vi "TCS Command Test Program.vi"() -> ()   [LabVIEW 2022 SP3]
uses:
  typedefs/CC cluster Object.ctl
  typedefs/CC cluster sidereal rate.ctl
  typedefs/CC cluster RA and DEC.ctl
  typedefs/cc cluster muRA muDEC.ctl
  Telescope/CC cluster Telescope Offsets.ctl
  TCS/TCS_external_interfaces/TCSDataDefinitions/TCSCommand/TCSTcsCommand/TCSTcsCommand.lvclass
  TCS/TCS_external_interfaces/TCSDataDefinitions/TCSCommand/TargetConfiguration/Target/FixedTarget/RADecParameters/RADecParameters.lvclass
  TCS/TCS_external_interfaces/TCSDataDefinitions/TCSCommand/TargetConfiguration/Target/FixedTarget/Declination/Declination.lvclass
  TCS/TCS_external_interfaces/TCSDataDefinitions/TCSPublicStatus/CurrentTimes/ClockTimes/ClockTimes.lvclass
  TCS/TCS_external_interfaces/TCSDataDefinitions/TCSCommand/TargetConfiguration/ScienceTargetConfiguration/ScienceTargetConfiguration.lvclass
  C:/Development/TCS/TCS_external_interfaces/TCSDataDefinitions/TCSCommand/TargetConfiguration/TargetConfiguration/TargetConfiguration.lvclass
  TCS/TCS_external_interfaces/TCSDataDefinitions/TCSCommand/TargetConfiguration/Target/FixedTarget/RADecTarget/RADecTarget.lvclass
  C:/Development/TCS/TCS_external_interfaces/TCSDataDefinitions/TCSCommand/TargetConfiguration/Target/FixedTarget/FixedTarget/FixedTarget.lvclass
  C:/Development/TCS/TCS_external_interfaces/TCSDataDefinitions/TCSCommand/TargetConfiguration/Target/Target/Target.lvclass
  TCS/TCS_external_interfaces/TCSDataDefinitions/TCSCommand/TargetConfiguration/Target/FixedTarget/Declination/Declination.lvclass/Declination.ctl
  TCS/TCS_external_interfaces/TCSDataDefinitions/TCSPublicStatus/CurrentTimes/ClockTimes/ClockTimes.lvclass/ClockTimes.ctl
  TCS/TCS_external_interfaces/TCSDataDefinitions/TCSCommand/TargetConfiguration/Target/FixedTarget/RADecParameters/RADecParameters.lvclass/RADecParameters.ctl
  TCS/TCS_external_interfaces/TCSDataDefinitions/TCSCommand/TargetConfiguration/Target/FixedTarget/RADecTarget/RADecTarget.lvclass/RADecTarget.ctl
  TCS/TCS_external_interfaces/TCSDataDefinitions/TCSCommand/TargetConfiguration/Target/FixedTarget/FixedTarget/FixedTarget.lvclass/FixedTarget.ctl
  TCS/TCS_external_interfaces/TCSDataDefinitions/TCSCommand/TargetConfiguration/TargetConfiguration/TargetConfiguration.lvclass/TargetConfiguration.ctl
  TCS/TCS_external_interfaces/TCSDataDefinitions/TCSCommand/TargetConfiguration/TargetConfiguration/TargetConfiguration.lvclass
  TCS/TCS_external_interfaces/TCSDataDefinitions/TCSCommand/TargetConfiguration/Target/FixedTarget/FixedTarget/FixedTarget.lvclass
panel:
  out "XMLout":string
  out "XML out 2":string
  in  "Object out":T1
  in  "ClassLabel":string="TCSTcsCommand"
  out "XML out":string=" <target class=\"TCSDataDefinitions.TCSCommand.TargetConfiguration.Target.FixedTarget.RADecTarget\">\n  <commandID>100</commandID>\n  <tcsErrorResponse>\r\n    <status>false</status>\r\n    <code>0</code>\r\n    <source/>\r\n  </tcsErrorResponse>\n    <raDecParameters>\n      <declination>\n        <degreesDec>0</degreesDec>\n        <minutesArc>0</minutesArc>\n        <secondsArc>0</secondsArc>\n      </declination>\n      <equinoxPrefix>B</equinoxPrefix>\n      <equinoxYear>2000</equinoxYear>\n      <frame>FK4</frame>\n      <ra>\n        <hours>0</hours>\n        <minutesTime>0</minutesTime>\n        <secondsTime>0</secondsTime>\n      </ra>\n    </raDecParameters>\n    <parallax_Arcsec>0</parallax_Arcsec>\n    <properMotion>\n      <epochPM_Yr>2009</epochPM_Yr>\n      <pmdec_ArcsPYr>0</pmdec_ArcsPYr>\n      <pmra_SPYr>0</pmra_SPYr>\n    </properMotion>\n    <rv_kps>0</rv_kps>\n    <targetName>TargetName</targetName>\n    \n</target>\n"
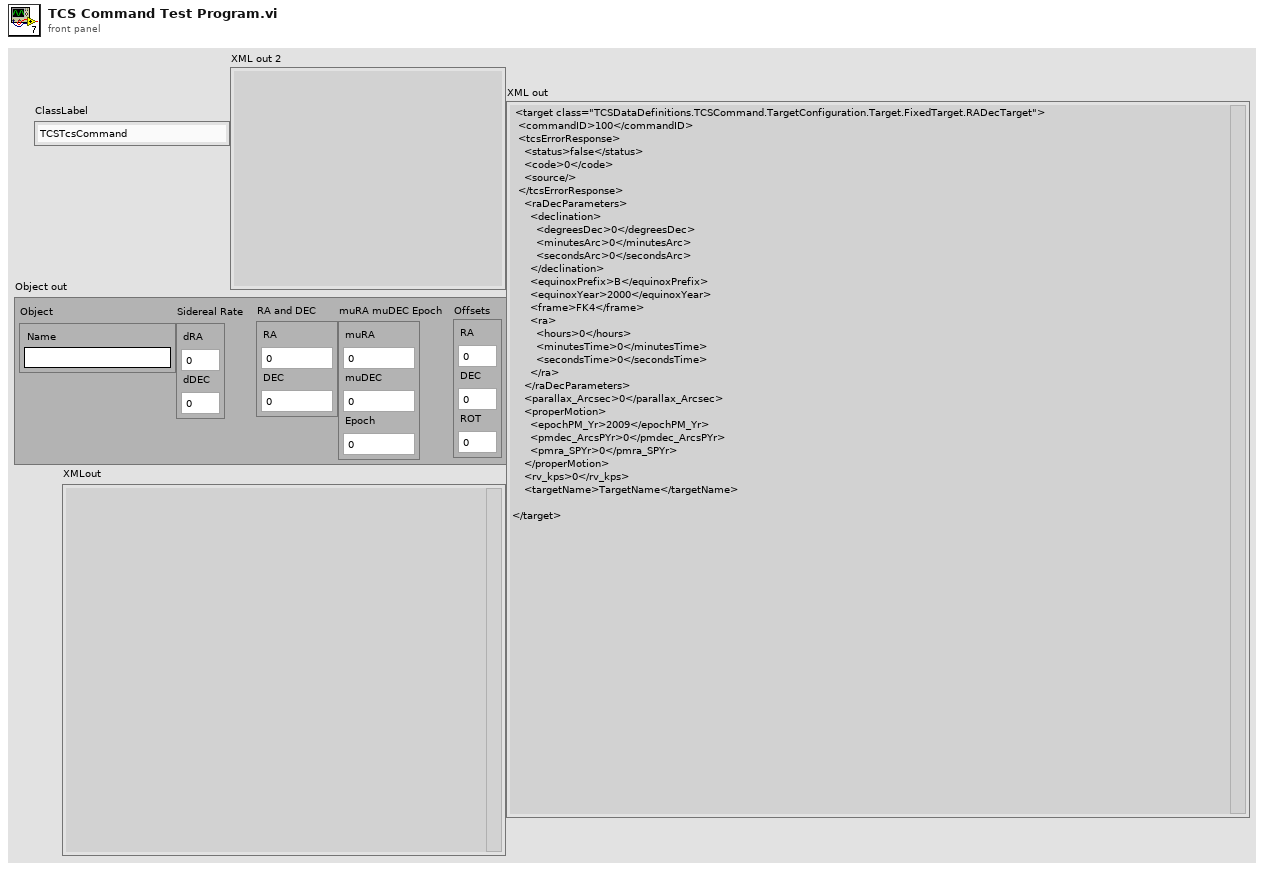
[diagram p1: front panel]
types:
  T1 = typedef "CC cluster Object.ctl" = cluster{"Object":cluster{"Name":string}, "Sidereal Rate":T2, "RA and DEC":T3, "muRA muDEC Epoch":T4, "Offsets":T5}
  T2 = typedef "CC cluster sidereal rate.ctl" = cluster{"dRA":dbl, "dDEC":dbl}
  T3 = typedef "CC cluster RA and DEC.ctl" = cluster{"RA":dbl, "DEC":dbl}
  T4 = typedef "cc cluster muRA muDEC.ctl" = cluster{"muRA":dbl, "muDEC":dbl, "Epoch":dbl}
  T5 = typedef "CC cluster Telescope Offsets.ctl" = cluster{"RA":dbl, "DEC":dbl, "ROT":dbl}
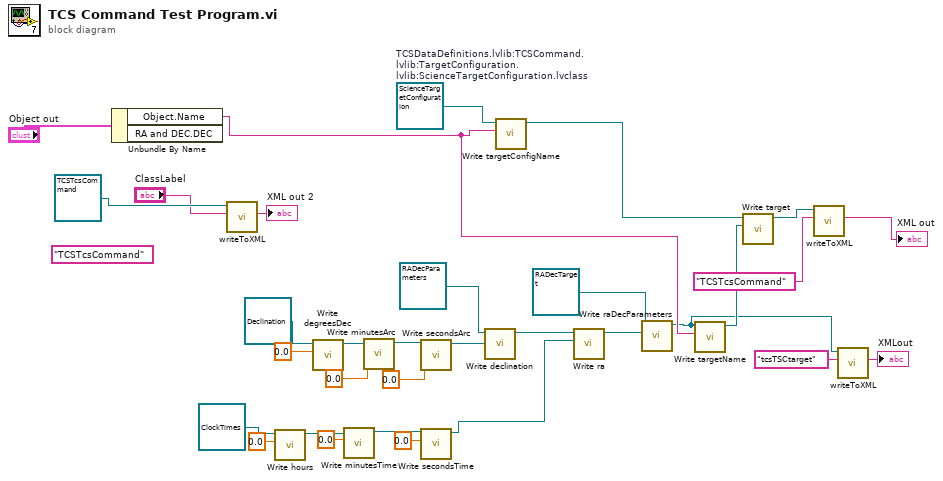
[diagram p0: block diagram]
diagram:
  (unwired) "TCSTcsCommand" ("ClassLabel")
  w11 = refnum<class "ScienceTargetConfiguration.lvclass"> refnum  # TCSDataDefinitions.lvlib:TCSCommand.lvlib:TargetConfiguration.lvlib:ScienceTargetConfiguration.lvclass
  n1 = Unbundle By Name("Object out") -> ("Object.Name"=w7:string)  [unwired: 1 out]
  n2 = call-dynamic "writeToXML.vi"("ClassLabel"="ClassLabel", "TCSTcsCommand in"=refnum<class "TCSTcsCommand.lvclass"> refnum ("TCSDataDefinitions.lvlib:TCSCommand.lvlib:TCSTcsCommand.lvclass")) -> ("XML out"=→"XML out 2":string)  [unwired: 7 in, 2 out]
  n3 = call "Write hours.vi"("hours"=dbl[unit] 0.0, "ClockTimes in"=refnum<class "ClockTimes.lvclass"> refnum ("ClockTimes.lvclass")) -> ("ClockTimes out"=w25:refnum<class "ClockTimes.lvclass">)  [unwired: 8 in, 1 out]
  n4 = call "Write degreesDec.vi"("degreesDec"=dbl[unit] 0.0, "Declination in"=refnum<class "Declination.lvclass"> refnum) -> ("Declination out"=w30:refnum<class "Declination.lvclass">)  [unwired: 8 in, 1 out]
  n5 = call "Write minutesTime.vi"("minutesTime"=dbl[unit] 0.0, "ClockTimes in"=w25) -> ("ClockTimes out"=w24:refnum<class "ClockTimes.lvclass">)  [unwired: 8 in, 1 out]
  n6 = call "Write minutesArc.vi"("minutesArc"=dbl[unit] 0.0, "Declination in"=w30) -> ("Declination out"=w29:refnum<class "Declination.lvclass">)  [unwired: 8 in, 1 out]
  n7 = call "Write secondsArc.vi"("secondsArc"=dbl[unit] 0.0, "Declination in"=w29) -> ("Declination out"=w28:refnum<class "Declination.lvclass">)  [unwired: 8 in, 1 out]
  n8 = call "Write secondsTime.vi"("secondsTime"=dbl[unit] 0.0, "ClockTimes in"=w24) -> ("ClockTimes out"=w21:refnum<class "ClockTimes.lvclass">)  [unwired: 8 in, 1 out]
  n9 = call "Write declination.vi"("Declination.lvclass"=w28, "RADecParameters in"=refnum<class "RADecParameters.lvclass"> refnum ("TCSDataDefinitions.lvlib:TCSCommand.lvlib:TargetConfiguration.lvlib:Target.lvlib:FixedTarget.lvlib:RADecParameters.lvclass")) -> ("RADecParameters out"=w22:refnum<class "RADecParameters.lvclass">)  [unwired: 8 in, 1 out]
  n10 = call "Write targetConfigName.vi"("targetConfigName"=w7, "TargetConfiguration in"=w11) -> ("TargetConfiguration out"=w10:refnum<class "ScienceTargetConfiguration.lvclass">)  [unwired: 8 in, 1 out]
  n11 = call "Write ra.vi"("ClockTimes.lvclass"=w21, "RADecParameters in"=w22) -> ("RADecParameters out"=w9:refnum<class "RADecParameters.lvclass">)  [unwired: 8 in, 1 out]
  n12 = call "Write raDecParameters.vi"("RADecParameters.lvclass"=w9, "RADecTarget in"=refnum<class "RADecTarget.lvclass"> refnum) -> ("RADecTarget out"=w2:refnum<class "RADecTarget.lvclass">)  [unwired: 8 in, 1 out]
  n13 = call "Write targetName.vi"("targetName"=w7, "FixedTarget in"=w2) -> ("FixedTarget out"=w8:refnum<class "RADecTarget.lvclass">)  [unwired: 8 in, 1 out]
  n14 = call "Write target.vi"("Target.lvclass"=w8, "TargetConfiguration in"=w10) -> ("TargetConfiguration out"=w3:refnum<class "ScienceTargetConfiguration.lvclass">)  [unwired: 8 in, 1 out]
  n15 = call-dynamic "writeToXML.vi"("ClassLabel"="TCSTcsCommand", "ScienceTargetConfiguration in"=w3) -> ("XML out"=→"XML out":string)  [unwired: 7 in, 2 out]
  n16 = call-dynamic "writeToXML.vi"("ClassLabel"="tcsTSCtarget", "RADecTarget in"=w2) -> ("XMLout"=→"XMLout":string)  [unwired: 7 in, 2 out]
